vi "Concatenate String Array.vi"(11 "Array":string[](array[string])) -> (3 "Concatenated String":string)   [LabVIEW 2018, in "Receipt Parsing.lvlib"]
uses:
  Receipt Parsing.lvlib
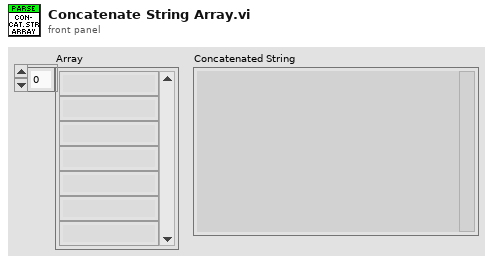
[diagram p1: front panel]
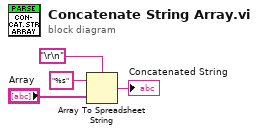
[diagram p0: block diagram]
diagram:
  n1 = Array To Spreadsheet String(delimiter (Tab)="\r\n", array="Array", 3:"%s" ("format string")) -> (spreadsheet string=→"Concatenated String":string)
